vi "LVCAM Read LVCAM.vi"(11 "LVCAM Read LVCAM in":refnum<class "LVCAM Read LVCAM.lvclass">) -> (2 "LVCAM":refnum<class "LVCAM.lvclass">)   [LabVIEW 2021, in "LVCAM.lvlib" / "LVCAM Read LVCAM.lvclass"]
uses:
  LVCAM Read LVCAM.lvclass
  LVCAM/LVCAM.lvclass
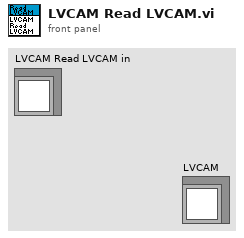
[diagram p1: front panel]
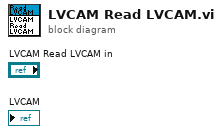
[diagram p0: block diagram]
diagram:
